vi "imagenCamSinGuardar.vi"(4 "Valor Gamma":dbl=1.0 min=1.0 max=2.2, 6 "Ganancia":i64 min=0 max=100, 7 "Exposure":dbl=0.05 min=5e-05 max=0.053229, 8 "tiempo de exposición (ms)":i32, 11 "Optional Rectangle":i32[](array[numeric])) -> (1 "Image Pixels (U8)":u8[][](array[numeric]), 2 "Image":T3(plugin-control))   [LabVIEW 2016]
uses:
  <vilib>/vision/driver/IMAQdx.llb/IMAQdx Attribute Type.ctl
  <vilib>/userdefined/High Color/IMAQdx.ctl
  <vilib>/Platform/TimedLoop/XDataNode/timing_clust.ctl
  <vilib>/Platform/TimedLoop/XDataNode/nitl_modes.ctl
  <vilib>/Platform/TimedLoop/XDataNode/wakeup.ctl
  <vilib>/platform/TimedLoop/XDataNode/XDataNode.xnode
  <vilib>/vision/driver/NI_Vision_Acquisition_Software.lvlib
  <vilib>/Platform/TimedLoop/XDataNode/XDNodeRunTimeDep.lvlib
  <resource>/objmgr/imaqdx.rc
  <vilib>/vision/NI_Vision_Development_Module.lvlib
panel:
  out "Attribute Information Array":T2(array[cluster])
  out "Image Pixels (U8) 2":u8[][](array[numeric])
  out "Image 2":T3(plugin-control)
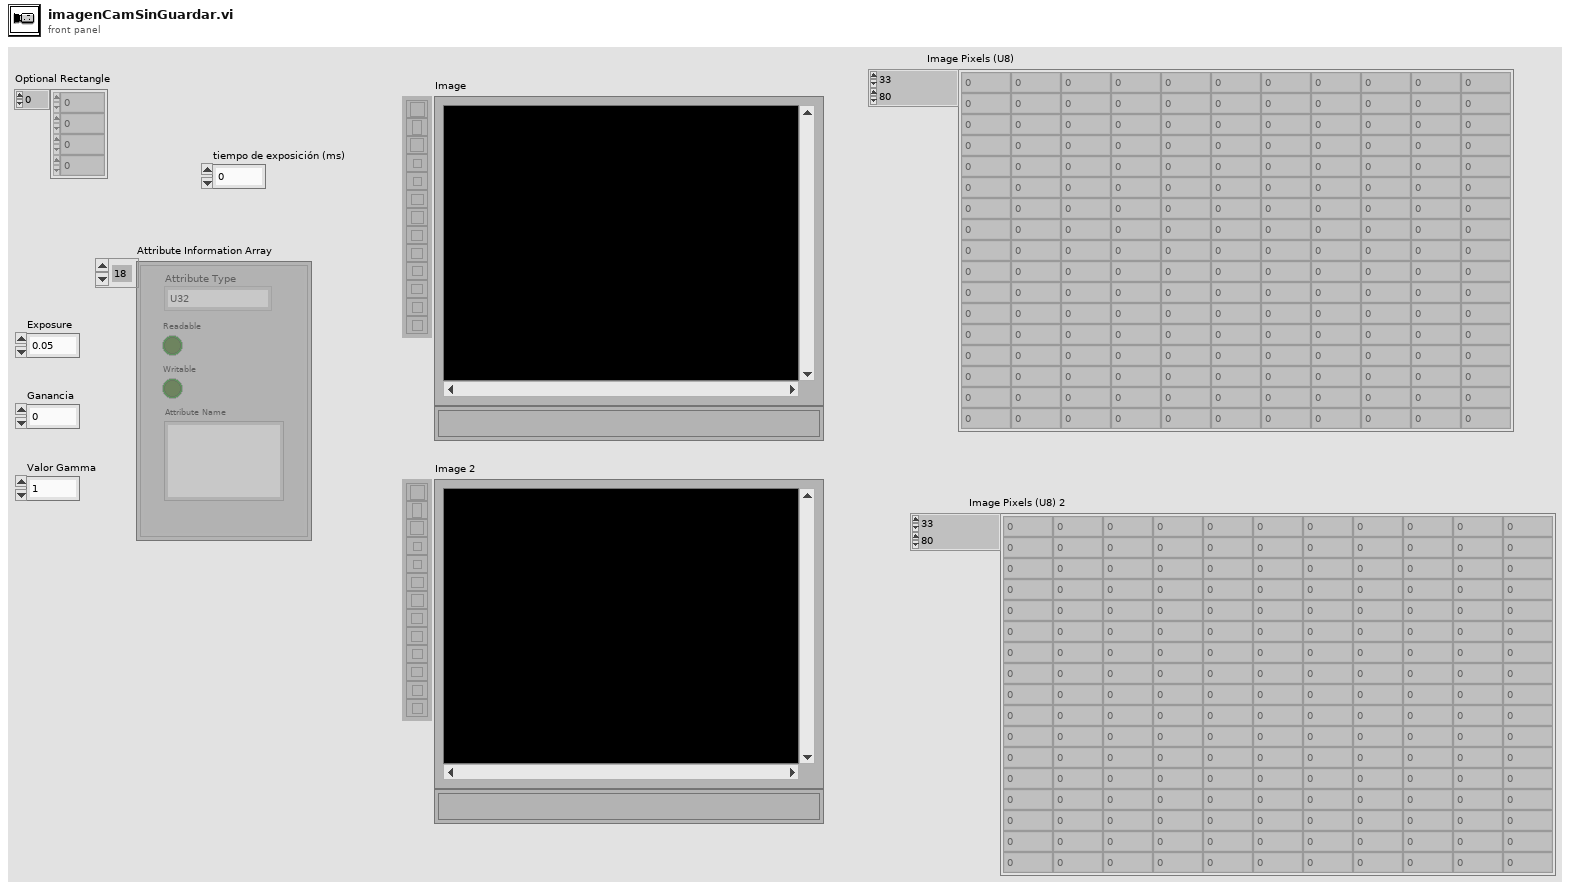
[diagram p1: front panel]
types:
  T1 = typedef "NI_Vision_Acquisition_Software.lvlib/IMAQdx Attribute Type.ctl" = enum32{"U32", "I64", "DBL", "String", "Enum", "Bool", "Command"}
  T2 = cluster{"Attribute Type":T1, "Readable":bool, "Writable":bool, "Attribute Name":string}[]
  T3 = typedef "IMAQ Image.ctl" = refnum<image>
  T4 = typedef "IMAQdx.ctl" = refnum<k21>
  T5 = typedef "XDNodeRunTimeDep.lvlib/timing_clust.ctl" = cluster{"Expected End [f-1]":u64, "Actual End [f-1]":u64, "Finished Late? [f-1]":bool, "Expected End [i-1]":u64, "Actual End [i-1]":u64, "Finished Late? [i-1]":bool, "Expected Start [i]":u64, "Actual Start [i]":u64, "Expected Start [f]":u64, "Actual Start [f]":u64, "Source Name":string, "Structure Name":string, "Period":i64, "Deadline":i64, "Offset":i64, "Start":i64, "Priority":i32, "Timeout":i32, "Mode":T6, "Wakeup Reason":T7, "Error":errorcluster, "Source Type":string, "Secondary Source Type":string, "Global End Time":u64, "Global Start Time":u64, "Frame Duration":u64, "Iteration Duration":u64, "Assigned CPU":i32, "I/O Scan Engine Mode":u32}
  T6 = typedef "XDNodeRunTimeDep.lvlib/nitl_modes.ctl" = enum32{"No Change", "Process missed periods, maintain original phase", "Discard missed periods, maintain original phase", "Process missed periods, ignore original phase", "Discard missed periods, ignore original phase"}
  T7 = typedef "XDNodeRunTimeDep.lvlib/wakeup.ctl" = enum32{"Normal", "Aborted", "Asynchronous wakeup", "Timing source error", "Timed loop error", "Timeout"}
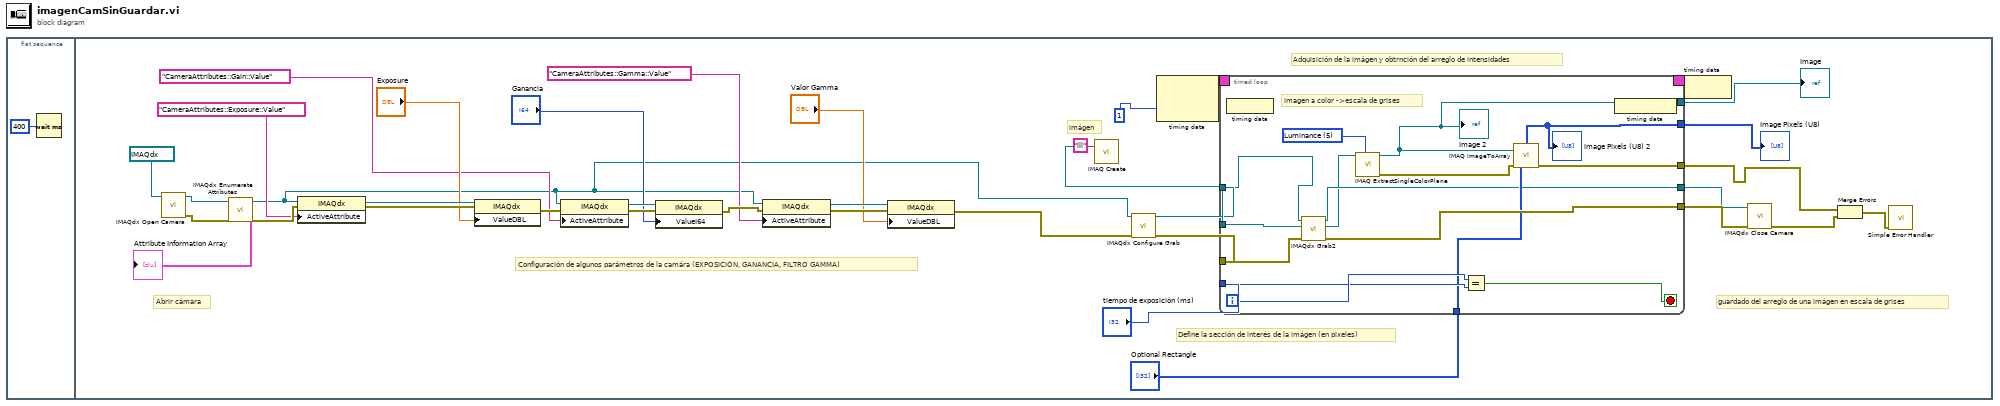
[diagram p0: block diagram]
diagram:
  n1 = flat-sequence {
    frame #0 {
      n2 = Wait (ms)(milliseconds to wait=u32 400) -> ()  [unwired: 1 out]
    }
    frame #1 {
      # "imágen"
      # "Define la sección de interés de la imágen (en pixeles)"
      # "Configuración de algunos parámetros de la camára (EXPOSICIÓN, GANANCIA, FILTRO GAMMA)"
      # "Abrir cámara"
      # "guardado del arreglo de una imágen en escala de grises"
      # "Adquisición de la imágen y obtrnción del arreglo de intensidades"
      n3 = call <vilib>:"IMAQdx Open Camera.vi"("Session In"=T4 "cam4") -> ("error out"=w22:errorcluster, "Session Out"=w3:T4)  [unwired: 9 in]
      n4 = call <vilib>:"IMAQdx Enumerate Attributes.vi"("error in"=w22, "Session In"=w3) -> ("error out"=w20:errorcluster, "Attribute Information Array"=→"Attribute Information Array":T2, "Session Out"=w4:T4)  [unwired: 7 in]
      n5 = property class="IMAQdx"(reference=w4, error in=w20, "ActiveAttribute"="CameraAttributes::Exposure::Value") -> (reference out=w17:T4, error out=w18:errorcluster)
      n6 = property class="IMAQdx"(reference=w17, error in=w18, "ValueDBL"="Exposure") -> (error out=w15:errorcluster)  [unwired: 1 out]
      n7 = property class="IMAQdx"(reference=w4, error in=w15, "ActiveAttribute"="CameraAttributes::Gain::Value") -> (reference out=w13:T4, error out=w12:errorcluster)
      n8 = property class="IMAQdx"(reference=w13, error in=w12, "ValueI64"="Ganancia") -> (error out=w8:errorcluster)  [unwired: 1 out]
      n9 = property class="IMAQdx"(reference=w4, error in=w8, "ActiveAttribute"="CameraAttributes::Gamma::Value") -> (reference out=w10:T4, error out=w9:errorcluster)
      n10 = property class="IMAQdx"(reference=w10, error in=w9, "ValueDBL"="Valor Gamma") -> (error out=w5:errorcluster)  [unwired: 1 out]
      n11 = call "IMAQ Create"("Image Name"="lll") -> ("New Image"=w36:T3)  [unwired: 4 in, 1 out]
      n12 = call <vilib>:"IMAQdx Configure Grab.vi"("error in"=w5, "Session In"=w4) -> ("error out"=w32:errorcluster, "Session Out"=w33:T4)  [unwired: 8 in]
      n13 = node-c288(i64 1 ("Period")) -> (w25:T5)  [unwired: 1 in]
      n14 = timed-loop {
        tunnel: w36 -> [w53]
        tunnel: [w52] -> w35
        tunnel: w33 -> [w43]
        tunnel: [w44] -> w34
        tunnel: w32 -> [w51]
        tunnel: "tiempo de exposición (ms)" -> [w49]
        tunnel: [w45] -> w2
        tunnel: "Optional Rectangle" -> [w47]
        tunnel: [w41] -> w29
        tunnel: [w46] -> w27
        timing: w25 -> [_]
        timing-out: [_] -> w24
        i -> [w50]
        stop <- w48 stop-if-true
        w40 = 5 items=["Red", "Green", "Blue", "Hue", "Saturation", "Luminance", "Value", "Intensity"] ("Color Plane")
        # "imagen a color ->escala de grises"
        n15 = node-c288() -> ()  [unwired: 1 in]
        n16 = call <vilib>:"IMAQdx Grab2.vi"("error in"=w51, "Image In"=w53, "Session In"=w43) -> ("error out"=w52:errorcluster, "Image Out"=w39:T3, "Session Out"=w44:T4)  [unwired: 5 in, 1 out]
        n17 = call "IMAQ ExtractSingleColorPlane"("Color Plane"=w40, "Image Src"=w39) -> ("error out"=w42:errorcluster, "Image Dst Out"=w41:T3)  [unwired: 8 in]
        "Image 2" <- w41
        n18 = Equal?(x=w50, y=w49) -> (x = y?=w48:bool)
        n19 = call "IMAQ ImageToArray"("error in (no error)"=w42, "Optional Rectangle"=w47, "Image"=w41) -> ("error out"=w46:errorcluster, "Image Pixels (U8)"=w45:u8[][])  [unwired: 1 in, 3 out]
        "Image Pixels (U8) 2" <- w45
        n20 = node-c288() -> ()  [unwired: 1 out]
      }
      "Image Pixels (U8)" <- w2
      "Image" <- w29
      n21 = node-c288(w24) -> ()
      n22 = call <vilib>:"IMAQdx Close Camera.vi"("error in"=w35, "Session In"=w34) -> ("error out"=w26:errorcluster)  [unwired: 9 in]
      n23 = Merge Errors(w27, w26) -> (w28:errorcluster)
      n24 = call <vilib>:"Simple Error Handler.vi"("error in (no error)"=w28) -> ()  [unwired: 4 in, 5 out]
    }
  }
